vi "TCL Get Fragments - 1event1frag.vi"(0 "event file":path, 1 "event number":i32, 3 "primary key":string, 4 "fragment":string, 5 "error in (no error)":errorcluster) -> (6 "fragments out":string[](array[string]), 7 "values":string[][](array[string]), 8 "error out":errorcluster)   [LabVIEW 2010]
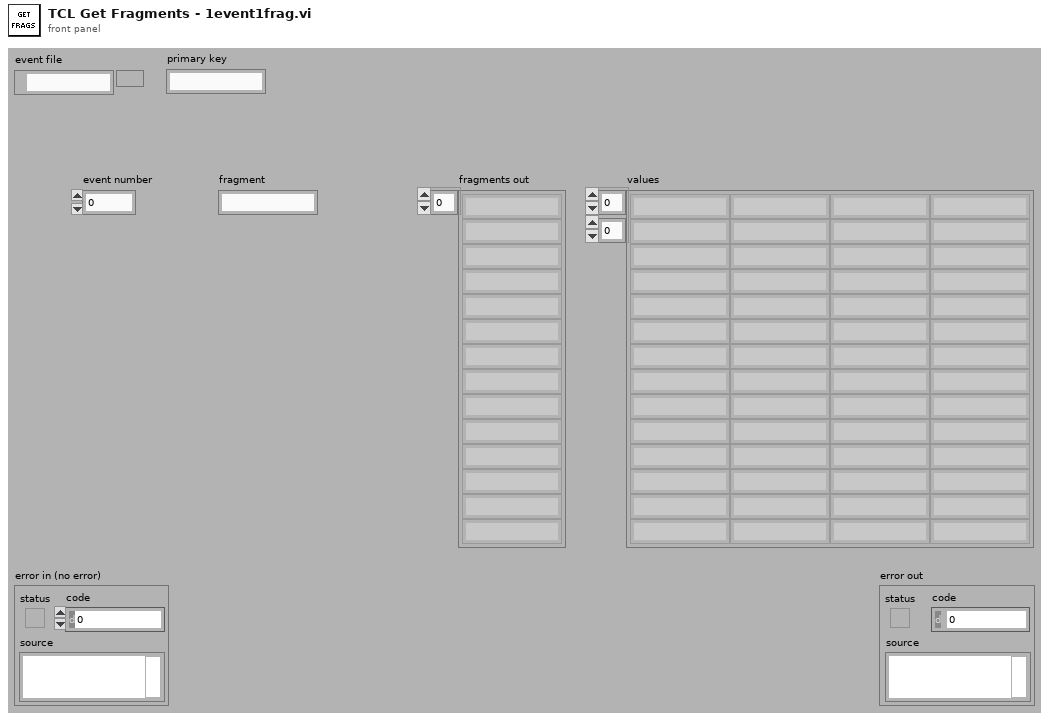
[diagram p1: front panel]
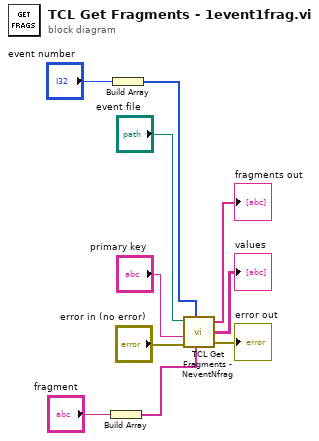
[diagram p0: block diagram]
diagram:
  n1 = Build Array("fragment") -> (w2:string[])
  n2 = Build Array("event number") -> (w10:i32[])
  n3 = call "TCL Get Fragments - NeventNfrag.vi"("event file"="event file", "event numbers"=w10, "primary key"="primary key", "fragments"=w2, "error in (no error)"="error in (no error)") -> ("fragments out"=→"fragments out":string[], "values"=→"values":string[][], "error out"=→"error out":errorcluster)  [unwired: 1 in]
